vi "NMRFMsweep.vi"(0 "Center Freq (MHz)":dbl=213.0, 2 "Freq Span (kHz)":dbl=2000.0, 3 "RF Level (dBm)":dbl, 4 "Program":bool, 7 "GPIB Addr (28)":refnum<visa-resource-name>="GPIB0::28::INSTR") -> (1 "error out":errorcluster)   [LabVIEW 2018]
uses:
  rssmt.llb/RS SMT Outputs On/Off.vi
panel:
  in  "Mod. Source (0:LFgen1)":i32(ring)=1 items=["LFgen1", "External1", "External2"]
  # "The big kahuna to setup the FM sweep\nand amplitude"
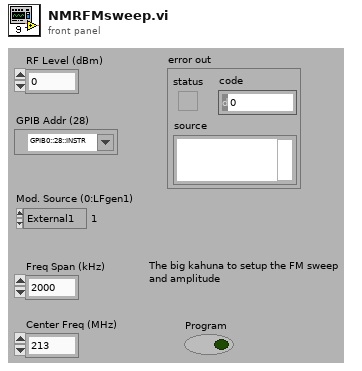
[diagram p1: front panel]
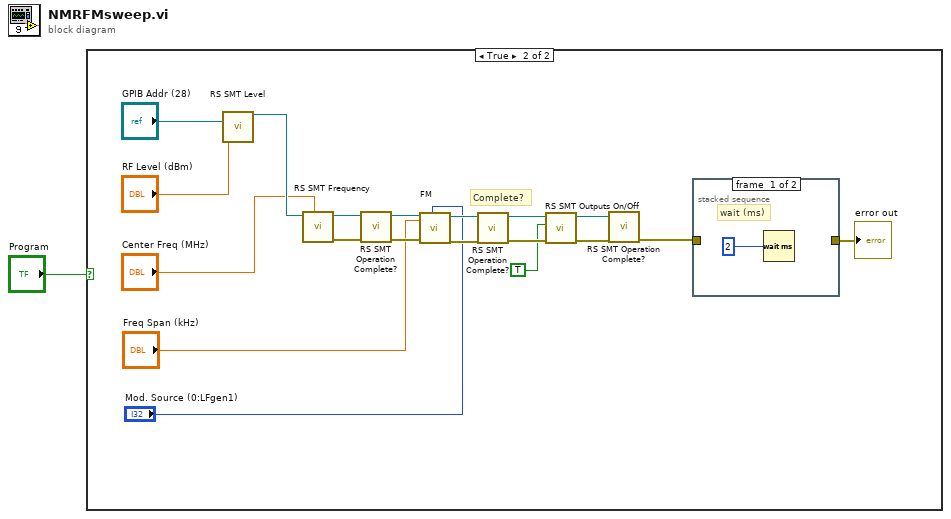
[diagram p0: block diagram]
diagram:
  n1 = case shown="True" "Program" {
    frame False {
    }
    frame True {
      # "Complete?"
      n2 = call "RS SMT Level.vi"("VISA session"="GPIB Addr (28)", "Level (-30.0)"="RF Level (dBm)") -> ("dup VISA session"=w17:refnum<visa-resource-name>)  [unwired: 12 in, 1 out]
      n3 = call "RS SMT Frequency.vi"("Frequency (100.0 MHz)"="Center Freq (MHz)", "VISA session"=w17) -> ("error out"=w15:errorcluster, "dup VISA session"=w16:refnum<visa-resource-name>)  [unwired: 8 in]
      n4 = call "RS SMT Operation Complete?.vi"("error in (no error)"=w15, "VISA session"=w16) -> ("error out"=w11:errorcluster, "dup VISA session"=w12:refnum<visa-resource-name>)  [unwired: 8 in]
      n5 = call "FM.vi"("VISA session"=w12, "Dev (10.0 kHz)"="Freq Span (kHz)", "error in (no error)"=w11, "Mod. Source (0:LFgen1)"="Mod. Source (0:LFgen1)") -> ("dup VISA session"=w13:refnum<visa-resource-name>, "error out"=w10:errorcluster)  [unwired: 14 in]
      n6 = call "RS SMT Operation Complete?.vi"("error in (no error)"=w10, "VISA session"=w13) -> ("error out"=w5:errorcluster, "dup VISA session"=w7:refnum<visa-resource-name>)  [unwired: 8 in]
      n7 = call "RS SMT Outputs On/Off.vi"("error in (no error)"=w5, "RF Output (F:Off)"=TRUE, "VISA session"=w7) -> ("error out"=w4:errorcluster, "dup VISA session"=w6:refnum<visa-resource-name>)  [unwired: 7 in]
      n8 = call "RS SMT Operation Complete?.vi"("error in (no error)"=w4, "VISA session"=w6) -> ("error out"=w3:errorcluster)  [unwired: 8 in, 1 out]
      n9 = stacked-sequence {
        tunnel: w3 -> [_ w22]
        tunnel: [_ w22] -> w18
        frame #0 {
          # "wait (ms)"
          n10 = Wait (ms)(milliseconds to wait=2) -> ()  [unwired: 1 out]
        }
        frame #1 {
        }
      }
      "error out" <- w18
    }
  }
